vi "Format_CMRR_BW.vi"(4 "Range Count":i32=12, 6 "First Range":i32, 9 "PSRR/CMRR/BW":T1={"Freq (Hz)"=[[0.0, 49.98779296875], [49.98779296875, 100.006103515625], [100.006103515625, 149.993896484375], [149.993896484375, 200.01220703125], [200.01220703125, 250.0], [0.0, 250.0], [49.98779296875, 100.006103515625]], "SNR (dBFS)"=[122.49294424672361, 122.35389846356063, 122.34393026582947, 122.45111299294416, 122.45121773152403, 115.43161378863995, 122.35389846356063], "Fund(dB)"=0.0}) -> (1 "CMRR/BW Table":string[][](table))   [LabVIEW 2010]
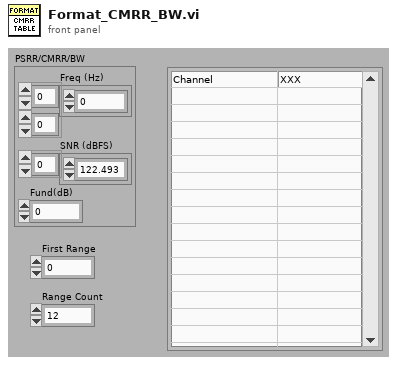
[diagram p1: front panel]
types:
  T1 = cluster{"Freq (Hz)":dbl[][], "SNR (dBFS)":dbl[], "Fund(dB)":dbl}
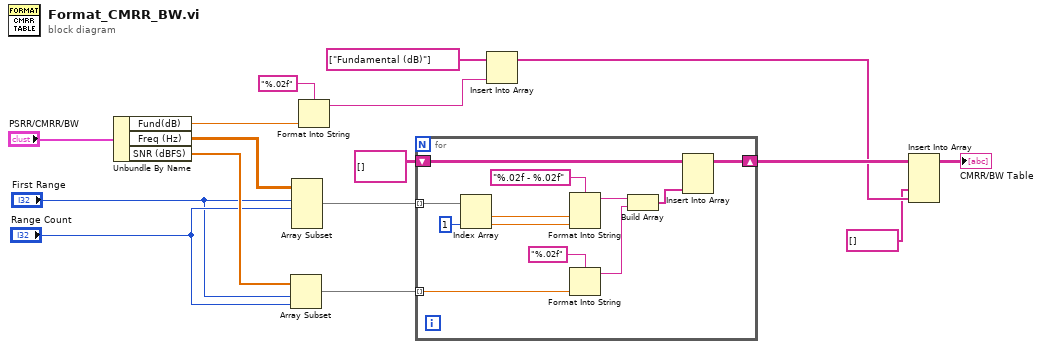
[diagram p0: block diagram]
diagram:
  n1 = Unbundle By Name("PSRR/CMRR/BW") -> ("Fund(dB)"=w14:dbl, "Freq (Hz)"=w6:dbl[][], "SNR (dBFS)"=w4:dbl[])
  n2 = Array Subset(array=w4, index="First Range", length="Range Count") -> (w3:dbl[])
  n3 = Array Subset(array=w6, index (row)="First Range", length (row)="Range Count") -> (w5:dbl[][])  [unwired: 2 in]
  n4 = Format Into String(format string="%.02f", w14) -> (resulting string=w9:string)  [unwired: 2 in, 1 out]
  n5 = for {
    tunnel: w5 -> [w27] mode=indexing
    tunnel: w3 -> [w23] mode=indexing
    shift-right: [w20] -> w13
    shift-left: string[][] [] -> [w21]
    n6 = Index Array(array=w27, index #2=1 ("index")) -> (element #1=w25:dbl, element #2=w24:dbl)  [unwired: 1 in]
    n7 = Format Into String(format string="%.02f - %.02f", w25, w24) -> (resulting string=w19:string)  [unwired: 2 in, 1 out]
    n8 = Format Into String(format string="%.02f", w23) -> (resulting string=w18:string)  [unwired: 2 in, 1 out]
    n9 = Build Array(w19, w18) -> (w17:string[])
    n10 = Insert Into Array(array=w21, new element=w17) -> (w20:string[][])  [unwired: 2 in]
  }
  n11 = Insert Into Array(array=string[] ["Fundamental (dB)"], new element=w9) -> (w8:string[])  [unwired: 1 in]
  n12 = Insert Into Array(array=w13, new element #1=string[] [] ("new element/subarray"), new element #2=w8) -> (→"CMRR/BW Table":string[][])  [unwired: 2 in]
